vi "AlliGator Send Plots to Image Profile Window.vi"(7 "Image Control Refnum":T2, 8 "error in (no error)":errorcluster, 9 "Fit Parameter":T1, 11 "AlliGator IV DVR in":refnum<data-value>) -> (0 "error out":errorcluster, 3 "AlliGator IV DVR out":refnum<data-value>)   [LabVIEW 2021, in "AlliGator Image Profile Window.lvlib"]
doc: "Computes plots and send them to the Profile Window."
uses:
  AlliGator Image Profile Window.lvlib
  Internal Variables/AlliGator Internal Variables v2.ctl
  <vilib>/vision/Image Controls.llb/IMAQ Image.ctl
  Internal Variables/AlliGator Gate Image Set.ctl
  Files/AlliGator FLI Dataset Type.ctl
  Files/AlliGator Data Series Type.ctl
  Dual-Channel Datasets/AlliGator Dataset Channel.ctl
  Settings/AlliGator Gate Arithmetic.ctl
  Source Image/AlliGator Displayed Image.ctl
  Image/Named ROI Description.ctl
  Phasor Graph/AlliGator Decay Metadata v3.ctl
  Decay Analysis/Decay Preprocessing/AlliGator Decay Background Subtraction Info.ctl
  Decay Analysis/Decay Preprocessing/AlliGator Baseline Subtraction Method.ctl
  Graphs/XY Graph/XY Graph Plot Shift Parameters.ctl
  Graphs/XY Graph/XY Graph Plot Shift Method.ctl
  Decay Analysis/Decay Preprocessing/AlliGator Decay Extrapolation Parameters.ctl
  Phasor/Calibration Phasor (m, phi).ctl
  Phasor/Phasor Reference Series.ctl
  Phasor/Phasor Calibration Map v2.ctl
  Phasor/Phasor (g, s).ctl
  Phasor Graph/AlliGator Raw Phasor Plot Data v5.ctl
  Phasor/Phasor Standard Deviation Options.ctl
  Phasor Plot/AlliGator Phasor Multi-Harmonic Data.ctl
  Phasor/Phasor Harmonic Data.ctl
  Decay Fit Parameter Map/AlliGator Decay Fit Options & Parameters v4.ctl
  Fits/IRF(X)PSED/Decay Fit Options v4.ctl
  Fits/Decay Convolution/Decay Model.ctl
  Fits/Residual Type.ctl
  Fits/IRF(X)PSED/Fit Weights Type v2.ctl
  Fits/Non-linear Fitting Method v2.ctl
  Fits/Fit Calculation Method.ctl
  Fits/Non-linear Fitting Algorithm.ctl
  Decay Analysis/Decay Fit/AlliGator Decay Fit Parameter Constraints 2.ctl
  Fits/IRF(X)PSED/Decay Fit Parameters In List.ctl
  Fits/IRF(X)PSED/MLE Baseline Offset Type.ctl
  Decay Analysis/Decay Preprocessing/AlliGator Decay Preprocessing Parameters.ctl
  Fits/IRF(X)PSED/Decay Fit Parameters & Derived Quantities List v2.ctl
  Fits/IRF(X)PSED/Decay Fit Result Constraint.ctl
  Decay Fit Parameter Map/AlliGator Parameter Maps Data.ctl
  Image/Image Control Refnum.ctl
  Globals, Variables, Constants/AlliGator Variables List.ctl
  Settings/AlliGator Settings List.ctl
  Image/Box Profile Type.ctl
  AlliGator Image Profile Average Intensity Type.ctl
  AlliGator Image Profile Intensity Type.ctl
  AlliGator Image Profile Data.ctl
  Image/Image ROI Type.ctl
  AlliGator Image Profile Plot Data.ctl
  Graphs/XY Graph/XY Graph Plot Data.ctl
  Phasor/Phasor Ratio Type.ctl
  Phasor Ratio/AlliGator Phasor Ratio Color-Coded Quantity.ctl
  Variant/Variant to Data/Variant to Boolean.vi
  Variant/Variant to Data/Variant to DBL.vi
  Variant/Variant to Data/Variant to U16.vi
  Globals, Variables, Constants/AlliGator Globals, Variables & Constants.lvlib
  Graphs/XY Graph/XY Graph Add-Ons.lvlib
  Image/Image.lvlib
  Settings/AlliGator Settings.lvlib
  Variant/Variant to Data/Variant to Data.lvlib
  Decay Fit Parameter Map/AlliGator Decay Fit Parameter Map.lvlib
  Phasor/Phasor.lvlib
  Phasor Ratio/AlliGator Phasor Ratio.lvlib
  Math/Math.lvlib
  Internal Variables/AlliGator Internal Variables.lvlib
  Files/AlliGator Files.lvlib
  Phasor Graph/AlliGator Phasor Graph.lvlib
  Decay Analysis/Decay Preprocessing/AlliGator Decay Preprocessing.lvlib
  Phasor Plot/AlliGator Phasor Plot.lvlib
  Source Image/AlliGator Source Image.lvlib
  Fits/Fits.lvlib
  Decay Analysis/Decay Fit/AlliGator Decay Fit.lvlib
  Dual-Channel Datasets/AlliGator Dual-Channel Datasets.lvlib
panel:
  # "see the AlliGator License on the block diagram (Ctrl+E or Window:Show Block Diagram)"
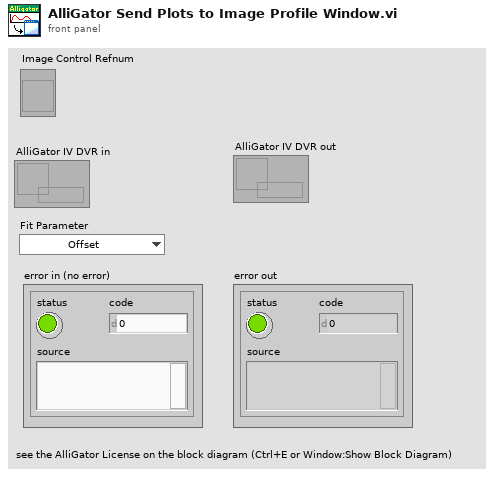
[diagram p1: front panel]
types:
  T1 = typedef "Fits.lvlib/Decay Fit Parameters & Derived Quantities List v2.ctl" = enum16{"Offset", "Baseline", "A_1", "tau_1", "A_2", "tau_2", "<tau>_a", "f1_a", "f2_a", "<tau>_i", "f1_i", "f2_i", "-", "R^2", "Chi^2"}
  T2 = typedef "Image.lvlib/Image Control Refnum.ctl" = refnum<vi>
  T3 = typedef "AlliGator Globals, Variables & Constants.lvlib/AlliGator Variables List.ctl" = enum16{"---- GUI ----", "GUI:Initialization Status", "GUI:State Indicators Refnum", "GUI:Original AlliGator Menu Items", "GUI:Current Action Loop State", "GUI:Script in progress", "GUI:Playback", "GUI:Loop Playback", "GUI:Search ROI Used", "GUI:Search ROI", "Decay Graph Max Legend Size", "Intensity Graph Max Legend Size", "Decay Statistics Graph Max Legend Size", "Phasor Graph Max Legend Size", "Phasor Ratio Graph Max Legend Size", "Lifetime Graph Max Legend Size", "---- Files ----", "Files:Export Dataset Frames as Individual Files", "Files:Show Batch Export Help Balloons", "Files:Frames in Dataset", "Files:ptu File Frame Start Indices", "Files:Current Frame in Dataset", "Files:Current Frame Timestamp", "Files:Dataset Loaded", "Files:Dataset Metadata", "Files:Dataset Channel", "Files:Dataset Data Description", "Files:Background Dataset Metadata", "Files:Background Dataset Channel", "Files:Background Dataset Data Description", "Files:Background File Subtraction", "Files:Background File Path", "Files:Background File Pile-up Correction", "Files:Background File Pixel Well Capacity", "Files:Background File Scaling Factor", "Files:Current Dataset Load Settings", "Files:Dataset Path", "Files:ICCD-specific Information", "Files:Macrotime Gate Separation", "------ Python Plugins ------", "Python Plugins:Information", "Python Plugins:Python Session", "Python Plugins:Valid Python Session?", "---- Source Image ----", "Source Image:ROIs", "Source Image:Current ROI", "Source Image:ROI Event Refnum", "X_Source Image:Display Range", "X_Source Image:Palette Information", "X_Source Image:Type of Displayed Image", "X_Time Gate Slider", "Source Image:Palette List", "Source Image:Scale", "Source Image:ROI Overlay Color", "Source Image:Overlay to Erase", "Source Image:Is Displayed Image Accumulated", "Source Image:White Light Image Modified", "Source Image:Mask Image Modified", "---- Image Profile Window ----", "Image Profile:Window Event Refnum", "Image Profile:IntensityType", "Image Profile:Intensity Average Type", "Image Profile:Intensity-weighted SDV", "Image Profile:Box Profile Type", "Image Profile:Window Open", "Image Profile:Plotted Fit Parameter", "------ Phasor Graph -------", "Phasor Graph:Show Line", "---- Phasor Plot ---", "Phasor Plot:Parameters Changed", "Phasor Plot:FLI Dataset Modified since last Calculation", "Phasor Harmonics Data", "Selected Phasor Harmonics", "Phasor Harmonic Manager Event Refnum", "Phasor Plot:ROIs", "Phasor Plot:Current ROI", "Phasor Plot:ROI Event Refnum", "Phasor Plot:Image Reference Points", "Phasor Plot:Computed", "Phasor Plot:Palette Information", "Phasor Plot:Palette List", "Phasor Plot:Phasor Ratio Palette Information", "Phasor Plot:Phasor Ratio Palette List", "Phasor Plot:Image Scale", "Phasor Plot:Image Overlay to Erase", "Phasor Plot:Image Elements to Update", "Phasor Plot:Current Calculation Parameters", "Phasor Plot:Current Calibration Options", "Phasor Plot:Reset Cumulated Phasor Plot", "Phasor Plot:Reference 1", "Phasor Plot:Lifetime Reference 1", "Phasor Plot:Reference 1 Frequency", "Phasor Plot:Reference 2", "Phasor Plot:Lifetime Reference 2", "Phasor Plot:Reference 2 Frequency", "---- Decay Analysis ----", "Number of Selected Decays to Fit", "LS Fit Results", "LAR Fit Results", "BS Fit Results", "Last Decay Max - Min", "Best Fit Parameters", "Best Fit Parameter Names", "Actual Size X", "Actual Size Y", "Binning X", "Binning Y", "Actual # Gates", "Dataset Number", "Gates to...", "Gates Skipped", "Gates to keep", "Gate Step", "Gate Separation", "Reversed Gates", "Pile-up Correction", "Pixel Well Capacity", "Background Subtracted", "Background Subtraction Method", "Background Definition Range", "Background File (deprecated)", "Number of Dataset Accumulated", "Array of Accumulated Dataset Paths", "Do Averaged Datasets", "Destination File Path", "Process Plot Target", "Use 1/D as Phasor Frequency", "---- Decay Fit Parameter Map -----", "Decay Fit Parameter Map:Palette Information", "Decay Fit Parameter Map:Palette List", "Decay Fit Parameter Map:X Resolution", "Decay Fit Parameter Map:Y Resolution", "Decay Fit Parameter Map:Use Decay Fit Result Constraints", "Decay Fit Parameter Map:Decay Fit Result Constraints", "Decay Fit Parameter Map:Decay Fit Result Constraints Applied", "---- Parameter Map ----", "Parameter Map:Palette Information", "Parameter Map:Palette List", "------- Local Decay Window ---------", "Local Decay Graph Window:Event Refnum", "Local Decay Graph Window:Use normalized IRF for convolution", "----- Miscellaneous ----", "Misc:Skippable Dialog Windows Status"}
  T4 = typedef "AlliGator Image Profile Window.lvlib/AlliGator Image Profile Intensity Type.ctl" = enum16{"Raw Data", "Displayed Image", "Background-subtracted"}
  T5 = typedef "AlliGator Image Profile Window.lvlib/AlliGator Image Profile Average Intensity Type.ctl" = enum16{"Integrated Intensity", "Average Intensity", "Intensity-weighted Average Intensity"}
  T6 = typedef "Image.lvlib/Box Profile Type.ctl" = enum16{"Full Width", "Half Width"}
  T7 = typedef "AlliGator Settings.lvlib/AlliGator Settings List.ctl" = enum16{"GUI:Visible Settings Tab", "GUI:Last Run Version", "Source Image:Use Image Histogram for Contrast", "Source Image:Low Count Pixels Rejection Options", "Source Image:High Count Pixels Rejection Options", "Source Image:Use Image Brightness", "Source Image:Blend Overlay with Image Background", "Source Image:Use Fixed ROI Diameter", "Source Image:ROI Diameter", "Source Image:ROI Center Color", "Source Image:Peak Threshold", "Source Image:Intensity Threshold", "Source Image:Image Binning Options", "Source Image:Image Smoothing Options", "Source Image:Image Histogram Active", "Source Image:Invert Binary Mask", "Source Image:Hot Pixel Removal", "Source Image:Overlay Analyzed ROI Center", "Source Image:Auto-Adjust Contrast", "Source Image:Histogram Lower Percentile", "Source Image:Histogram Upper Percentile", "Source Image:Save Source Image", "Source Image:Scale Bar Options", "Source Image:Image Resolution (Pixel Size)", "Source Image:Flatfield Correction", "Source Image:Show Dead Left Columns Correction", "Source Image:Dead Left Columns Correction", "Source Image:Image Pre-Processing Operations Order", "Source Image:Overlay ROI Median", "Source Image:Median Overlay Color", "Data Information:Gate Width", "Data Information:Nanotime Gate Separation", "Data Information:Macrotime Gate Separation", "Data Information:Gate Step", "Data Information:# Gates", "Data Information:Gate Image Exposure", "Data Information:Gate Image Integration", "Data Information:Gates to Skip", "Data Information:Gates to Keep", "Data Information:Define Gates to", "Data Information:Channel Name", "Data Information:Available Channel Names", "Data Information:Channel Arithmetic", "Data Information:Background File Subtraction", "Data Information:Background File", "Data Information:Background Scaling Factor", "Data Information:Background Pile-up Correction", "Data Information:Background Pixel Well Capacity", "Data Information:Laser Period", "Data Information:SYNC Period", "Data Information:Pile-up Correction", "Data Information:Pixel Well Capacity", "Data Information:Dataset Scaling Factor", "Fluorescence Decay_Decay Pre-Processing:Reverse Gates", "Fluorescence Decay_Decay Pre-Processing:Verbose Decay Pre-Processing", "Fluorescence Decay_Decay Pre-Processing:Use Decay Pre-Processing", "Fluorescence Decay_Decay Pre-Processing:Background Subtraction", "Fluorescence Decay_Decay Pre-Processing:Background Definition Range", "Fluorescence Decay_Decay Pre-Processing:Baseline Subtraction Method", "Fluorescence Decay_Decay Pre-Processing:Decay Pre-Processing Operations Order", "Fluorescence Decay_Decay Pre-Processing:Smoothing Parameter", "Fluorescence Decay_Decay Pre-Processing:Shift Decay", "Fluorescence Decay_Decay Pre-Processing:Decay Shift Parameters", "Fluorescence Decay_Decay Pre-Processing:Fold Decay", "Fluorescence Decay_Decay Pre-Processing:# Folds", "Fluorescence Decay_Decay Pre-Processing:1-Normalize Decay", "Fluorescence Decay_Decay Pre-Processing:[0-1]-Normalize Decay", "Fluorescence Decay_Decay Pre-Processing:Smoothen Decay", "Fluorescence Decay_Decay Pre-Processing:Extrapolate Decay", "Fluorescence Decay_Decay Pre-Processing:Use Periodicity", "Fluorescence Decay_Decay Pre-Processing:Use Cursors", "Fluorescence Decay_Decay Pre-Processing:Tail Fraction", "Fluorescence Decay_Decay Pre-Processing:Head Fraction", "Fluorescence Decay_Decay Pre-Processing:Additional Points", "Fluorescence Decay_Decay Pre-Processing:Straighten Decay", "Fluorescence Decay_Decay Pre-Processing:Constant Background", "Fluorescence Decay_Decay Pre-Processing:Pixel-Normalize Decay", "Fluorescence Decay_Advanced Analysis:Extract IRF instead of Decay", "Fluorescence Decay_Advanced Analysis:IRF Extraction Options", "Fluorescence Decay_Advanced Analysis:IRF Optimization Options", "Fluorescence Decay_Advanced Analysis:Square Pulse Options", "Fluorescence Decay_Advanced Analysis:IRF Order", "Fluorescence Decay_Advanced Analysis:IRF Time Constants", "Fluorescence Decay_Advanced Analysis:Wavelet Analysis Options", "Fluorescence Decay_Advanced Analysis:Average Lifetime Options", "Fluorescence Decay_Fit Options:Fit Options", "Fluorescence Decay_Fit Options:Use Legacy Fitting Approach", "Fluorescence Decay_Fit Options:Use Data Information Laser Period", "Fluorescence Decay_Fit Parameters:Displayed Fit Parameters", "Fluorescence Decay_Fit Parameters:Fit Parameter Constraints", "Fluorescence Decay_Fit Parameters:Export Tabulated Results", "Fluorescence Decay_Fit Parameters:MLE Baseline Offset Type", "Fluorescence Decay_Fit Parameters:MLE Baseline Offset", "Fluorescence Decay_Fit Parameters:Guess Parameter Names", "Fluorescence Decay_Fit Parameters:Guess Parameter Values", "Fluorescence Decay_Fit Parameters:Guess Parameters Options", "Fluorescence Decay_Fit Parameters:Optimal Offset Selection Criterion", "Fluorescence Decay_Styles:Show Last Decay Only", "Fluorescence Decay_Styles:Decay Graph Color Array", "Fluorescence Decay:Decay Graph Active", "Fluorescence Decay Statistics:Min Peak Value", "Fluorescence Decay Statistics:Reject Low Decay Peak Pixels", "Fluorescence Decay Statistics:Reject High Decay Peak Pixels", "Fluorescence Decay Statistics:Max Peak Value", "Time Traces:Use File Timestamp", "Time Traces:Time Step", "Time Traces:Use Intensity Correction File", "Time Traces:Intensity Correction File", "Phasor Plot:Phasor Plot Smoothing Options", "Phasor Plot:Phasor Plot Size", "Phasor Plot:Phasor Plot Graphics Options", "Phasor Plot:Cumulative Phasor Plot", "Phasor Plot:Use Phasor Brightness", "Phasor Plot:Blend Overlay with Phasor Background", "Phasor Plot:Save Phasor Plot", "Phasor Plot:Show References", "Phasor Plot:Phasor Ratio Decay Range", "Phasor Plot:Exponential Fading", "Phasor Plot:Phasor Ratio Reference Colors", "Phasor Plot:Reference Radius", "Phasor Plot:Show Color Map Vertices", "Phasor Plot:Phasor Plot Active", "Phasor Plot:Phasor Ratio Color Map Type", "Phasor Plot:Phasor Ratio Color Map", "Phasor Plot:Phasor Ratio Display Range", "Phasor Plot:Selected Image ROI(s)", "Phasor Plot:All Image ROIs", "Phasor Plot:Selected Phasor Plot ROI(s)", "Phasor Plot:All Phasor Plot ROIs", "Phasor Plot:Phasor Ratio Color-Coded Quantity", "Phasor Plot:Store Phasor Harmonics", "Phasor Plot:Draw Reference Segment", "Phasor Plot:User-Defined Quantity", "Phasor Plot:Color Scale High Color", "Phasor Plot:Color Scale Low Color", "Phasor Plot:Intensity-weighted Phasor Plot", "Phasor Graph:Phasor Frequency", "Phasor Graph:Phasor Ratio Type", "Phasor Graph:Pixel-level Phasor Computation", "Phasor Graph:Save Phasor Graph", "Phasor Graph:Phasor Graph Active", "Phasor Graph:Phasor SDV Options", "Phasor Graph:Intensity-weighted Phasor Graph", "Phasor Graph:Define Shortest Lifetime as", "Phasor Calibration:Use Backup Calibration if needed", "Phasor Calibration:Backup Calibration Type", "Phasor Calibration:Calibration Type", "Phasor Calibration:Calibration Lifetime", "Phasor Calibration:Calibration Map Algorithm", "Single-Exponential Phasor Locus (SEPL):Gate Parameters", "Single-Exponential Phasor Locus (SEPL):User-defined Gate", "Single-Exponential Phasor Locus (SEPL):User-defined IRF", "Single-Exponential Phasor Locus (SEPL):Phasor Parameters", "Single-Exponential Phasor Locus (SEPL):Decay & IRF Parameters", "Single-Exponential Phasor Locus (SEPL):Display Parameters", "Lifetime Analysis:Decay Analysis Parameters", "Lifetime Analysis:Lifetime Map Active", "Plugins:Python Settings", "Miscellaneous:Verbose Mode", "Miscellaneous:Beep after Script", "Miscellaneous:Saved Image File Format", "Miscellaneous:Exported Gate Image Settings", "Miscellaneous:Include Loading in Timing", "Miscellaneous:Verbose Settings Mode", "Miscellaneous:Histogram Options", "Miscellaneous:Beep on Error", "Miscellaneous:# Logical Processors Used", "Miscellaneous:ROI Description Max Characters", "Miscellaneous:Verbose Error Mode", "Miscellaneous:Transparent Mask Color"}
  T8 = typedef "AlliGator Image Profile Window.lvlib/AlliGator Image Profile Data.ctl" = cluster{"ROI Type":T9, "End Points":cluster{"X":dbl, "Y":dbl}[], "Profile Data":T10[]}
  T9 = typedef "Image.lvlib/Image ROI Type.ctl" = enum16{"No Selection", "Point", "Line", "Rectangle", "Oval", "Polygon", "Freehand Region", "Annulus", "Unused2", "Unused3", "Broken Line", "Freehand Line", "Rotated Rectangle"}
  T10 = typedef "AlliGator Image Profile Window.lvlib/AlliGator Image Profile Plot Data.ctl" = cluster{"Plot Name":string, "Plot":T11}
  T11 = typedef "XY Graph Add-Ons.lvlib/XY Graph Plot Data.ctl" = cluster{"X Array":dbl[], "Y Array":dbl[]}
  T12 = typedef "AlliGator Phasor Ratio.lvlib/AlliGator Phasor Ratio Color-Coded Quantity.ctl" = enum16{"Phasor Ratio (f1 or a1)", "Average Lifetime (<tau>_i or <tau>_a))", "User-Defined Quantity"}
  T13 = typedef "Phasor.lvlib/Phasor Ratio Type.ctl" = enum32{"Intensity-weighted", "Amplitude-weighted"}
  T14 = typedef "AlliGator Internal Variables.lvlib/AlliGator Internal Variables v2.ctl" = cluster{"----------------------------- Images -----------------------------":u8, "Displayed Image":T15, "White Light Image":T15, "Mask Image":T15, "ROI Mask Image":T15, "Current Dataset Images 1":T16, "Background Dataset Images 1":T16, "Current Dataset Images 2":T16, "Background Dataset Images 2":T16, "Current Dataset Arithmetic Images":T16, "Accumulated Dataset Images 1":T16, "Accumulated Dataset Images 2":T16, "Accumulated Dataset Arithmetic Images":T16, "----------------------------- File Paths -----------------------------":u8, "Phasor Plot Image":T15, "Decay Fit Parameter Map Image":T15, "Parameter Map Image":T15, "Single Data Point Path":path, "White Light Image Path":path, "Mask Image Path":path, "Time-Series Folder":path, "[Time-Series Paths]":path[], "----------------------------- FLI Dataset -----------------------------":u8, "Current Dataset":i32, "Single Dataset Type":T17, "Current Folder":string, "AlliGator Data Series Type":T18, "# Datasets":i32, "Dual-Channel Dataset":bool, "Selected Channel Name":string, "Dataset Channel":T19, "Channel Arithmetic":T20, "Dual-Channel Background Dataset":bool, "Background Channel":T19, "Dual-Channel Accumulated Dataset":bool, "Start Time":dbl, "[Time-Series Timestamps]":dbl[], "[Intensity Corrections]":dbl[], "Time Series Script":bool, "Type of Displayed Image":T21, "Gate Image Slide":u16, "# Gates":i32, "ROIs":T22[], "----------------------------- Decays -----------------------------":u8, "ROI Decay":cluster{"t Array":dbl[], "I Array":dbl[]}, "Valid Decay":bool, "Decay  Metadata":T24, "Reference Decay Plot Name":string, "Reference Decay":cluster{"t Array":dbl[], "I Array":dbl[]}, "Decay Shift Plot":cluster{"Time Stamps":dbl[], "Decay Shifts":dbl[]}, "[Decays Max Values]":sgl[], "[Decays Min Values]":sgl[], "----------------------------- Calibration -----------------------------":u8, "Calibration Phasor":T30, "Calibration Phasor Series":T31, "Phasor Calibration Map":T32, "Calibration Map MD5 Digest":string, "----------------------------- Phasor Graph -----------------------------":u8, "Last Raw Phasor":T33, "Last Calibrated Phasor":T33, "Last Calibrated Phasor SDV":T33, "Phasor Graph:Phasor Plot":cluster{"g Array":dbl[], "s Array":dbl[]}, "Phasor Graph:Phasor SDV Plot":cluster{"g Array":dbl[], "s Array":dbl[]}, "[Phasor Graph:Raw Phasor Plots]":T34[], "Phasor Plot locked to Ref 1":i32, "[Phasor Plot(s) locked to Ref 1]":i32[], "[Phasor Plot(s) locked to Ref 2]":i32[], "[Pixel Phasors]":T33[], "----------------------------- Phasor Plot -----------------------------":u8, "[[Sum Image]]":dbl[][], "[[CSG Phasors]]":csg[][], "[[Valid Pixel?]]":bool[][], "[[Phasor Ratios]]":dbl[][], "[[Average Lifetimes]]":dbl[][], "Amplitude Weighted Average Lifetime":bool, "I/m/phi Dataset":cluster{"I/m/phi Dataset?":bool, "Base Frequency":dbl[unit], "Harmonic Orders":u8[]}, "Multi Phasor Plot Data":T36, "----------------------------- Decay Fit Parameter Map -----------------------------":u8, "Decay Fit Options & Parameters":T38, "Fit Options: Decay Preprocessing Parameters":T49, "Fit Options: Reference Decay":cluster{"t Array":dbl[], "I Array":dbl[]}, "Is Full Image Parameters Map":bool, "Is Single-Pixels Parameters Map":bool, "NLSF Parameters Map X Resolution":i32, "NLSF Parameters Map Y Resolution":i32, "[Single Decay Fit Parameters]":dbl[], "Fit Model":T40, "[[Multiple Decays Fit Parameters]]":dbl[][], "[[Multiple Decays Fit Parameter SDVs]]":dbl[][], "[[IRFs]]":dbl[][], "[ROI Descriptors]":T23[], "IRF Array Time Axis":dbl[], "Decay Array Time Axis":dbl[], "[Decay Fit Parameter Names]":T1[], "[Decay Sum]":dbl[], "Array of Decay Fit Result Constraints":T50[], "Selected ROIs Array":bool[], "----------------------------- Parameter Maps -----------------------------":u8, "[Map Set Names]":string[], "[Parameter Maps]":T51[], "[[User-defined Quantities]]":dbl[][], "User-defined Quantity":string}
  T15 = typedef "IMAQ Image.ctl" = refnum<image>
  T16 = typedef "AlliGator Internal Variables.lvlib/AlliGator Gate Image Set.ctl" = cluster{"SGL Gate Images":T15[], "SGL Sum Image":T15, "SGL Max Image":T15, "SGL Min Image":T15}
  T17 = typedef "AlliGator Files.lvlib/AlliGator FLI Dataset Type.ctl" = enum16{"HDF5 FLI Dataset", "Gate Image Folder", ".sdt FLI Dataset (Becker & Hickl)", ".ptu FLI Dataset (PicoQuant)", "SS1 FLI Dataset", "SS2 FLI Dataset", "I/m/phi Dataset", ".bin FLI Dataset (PicoQuant Binned)", ".bin FLI Dataset (Piccolo Binned)", ".mat FLI Dataset"}
  T18 = typedef "AlliGator Files.lvlib/AlliGator Data Series Type.ctl" = enum16{"Not a Supported Series", "Gate Images Folder Series", "SwissSPAD 2 Dataset Series", "B&H FLI Dataset Series", "PicoQuant PTU FLI Dataset Series", "PicoQuant BIN FLI Dataset Series", "Piccolo hist BIN FLI Dataset Series", "HDF5 FLI Dataset Series"}
  T19 = typedef "AlliGator Dual-Channel Datasets.lvlib/AlliGator Dataset Channel.ctl" = enum16{"G2", "INT"}
  T20 = typedef "AlliGator Settings.lvlib/AlliGator Gate Arithmetic.ctl" = enum16{"None", "INT-G2", "G2/INT*<INT>", "(1 - G2/INT)*<INT>"}
  T21 = typedef "AlliGator Source Image.lvlib/AlliGator Displayed Image.ctl" = enum16{"Single Gate", "Sum of All Gates", "Max of All Gates", "Min of All Gates", "-", "White Ligth Image", "Mask Image"}
  T22 = typedef "Image.lvlib/Named ROI Description.ctl" = cluster{"ROI Descriptor":T23, "ROI Name":string, "Overlay Color":u32}
  T23 = typedef "ROI Descriptor" = cluster{"Global Rectangle":i32[], "Contours":cluster{"ID":enum32{"External", "Internal"}, "Type":u32, "Coordinates":i32[]}[]}
  T24 = typedef "AlliGator Phasor Graph.lvlib/AlliGator Decay Metadata v3.ctl" = cluster{"ROI Descriptor":T23, "ROI Center":cluster{"X":i32, "Y":i32}, "Decay Background Subtraction Info":T25, "Decay Reverted":bool, "Decay Smoothened":bool, "Decay Straightened":bool, "Fitted Tau (Decay Straightening)":dbl, "Decay Shift Parameters":T27, "Decay Shifted":bool, "Decay Extrapolated":bool, "Decay Extrapolation Parameters":T29, "Decay Normalized":bool, "Fold Decay":bool, "# Folds":u32}
  T25 = typedef "AlliGator Decay Preprocessing.lvlib/AlliGator Decay Background Subtraction Info.ctl" = cluster{"Laser Period":dbl[unit], "Gate Duration":dbl[unit], "Baseline Subtraction Method":T26, "Background Definition Range":cluster{"Min Gate":dbl[unit], "Max Gate":dbl[unit]}, "Total Intensity w/o Bkgd Subtraction":dbl, "Bkgd-subtracted Intensity (exp)":dbl, "# Data Points":i32, "Background/Gate":dbl, "Fitted Lifetime":dbl[unit], "Bkgd-subtracted Intensity (theo)":dbl}
  T26 = typedef "AlliGator Decay Preprocessing.lvlib/AlliGator Baseline Subtraction Method.ctl" = enum16{"Mean", "Min", "Square Gated Single-Exponential", "File", "Constant"}
  T27 = typedef "XY Graph Add-Ons.lvlib/XY Graph Plot Shift Parameters.ctl" = cluster{"Type":T28, "Shift":dbl[unit], "Threshold":dbl, "Rotate":bool}
  T28 = typedef "XY Graph Add-Ons.lvlib/XY Graph Plot Shift Method.ctl" = enum16{"Default", "CFD", "Threshold", "Cross-Correlation"}
  T29 = typedef "AlliGator Decay Preprocessing.lvlib/AlliGator Decay Extrapolation Parameters.ctl" = cluster{"Additional Points":u32, "Head Fraction":dbl, "Fitted Tau":dbl, "Use Periodicity":bool, "Use Cursors":bool, "Tail Fraction":dbl}
  T30 = typedef "Phasor.lvlib/Calibration Phasor (m, phi).ctl" = cluster{"m":dbl, "phi":dbl, "Phasor Frequency":dbl[unit], "Reference Lifetime":dbl[unit]}
  T31 = typedef "Phasor.lvlib/Phasor Reference Series.ctl" = cluster{"m Array":dbl[], "phi Array":dbl[], "Phasor Frequency":dbl[unit], "Calibration Lifetime":dbl[unit]}
  T32 = typedef "Phasor.lvlib/Phasor Calibration Map v2.ctl" = cluster{"Phasor Frequency":dbl[unit], "Calibration Lifetime":dbl[unit], "ROI Centers":cluster{"X":i32, "Y":i32}[], "ROI Descriptors":T23[], "Map Resolution X":i32, "Map Resolution Y":i32, "z Array":cdb[]}
  T33 = typedef "Phasor.lvlib/Phasor (g, s).ctl" = cluster{"g":dbl, "s":dbl}
  T34 = typedef "AlliGator Phasor Graph.lvlib/AlliGator Raw Phasor Plot Data v5.ctl" = cluster{"Phasor Plot Name":string, "Raw Phasor Plot":T33[], "Phasor Frequency":dbl[unit], "[Decay Metadata]":T24[], "Raw Phasor Plot SDV":T33[], "Phasor SDV Options":T35, "[Calibration Phasor]":T30[], "Intensity Array":dbl[]}
  T35 = typedef "Phasor.lvlib/Phasor Standard Deviation Options.ctl" = cluster{"Compute Estimated SDV":bool, "# Replicas":u32, "Use Estimated Average Phasor":bool}
  T36 = typedef "AlliGator Phasor Plot.lvlib/AlliGator Phasor Multi-Harmonic Data.ctl" = cluster{"Base Frequency":dbl[unit], "# Harmonics":u8, "Harmonic Orders":u8[], "Phasor Plot Settings Checksum":u64, "Phasor Harmonic Data Array":T37[]}
  T37 = typedef "Phasor.lvlib/Phasor Harmonic Data.ctl" = cluster{"Phasor Harmonic Name":string, "Phasor Plot Settings Checksum":u64, "Phasor Frequency":dbl[unit], "Base Frequency":dbl[unit], "Harmonic Order":u8, "Phasor Plot Parameters":string, "Phasor Array [[CSG]]":csg[][], "Dataset File Path":path}
  T38 = typedef "AlliGator Decay Fit Parameter Map.lvlib/AlliGator Decay Fit Options & Parameters v4.ctl" = cluster{"SYNC Period":dbl[unit], "Fit Options":T39, "Fit Parameter Constraints":T46[], "MLE Baseline Offset":dbl, "MLE Baseline Offset Type":T48}
  T39 = typedef "Fits.lvlib/Decay Fit Options v4.ctl" = cluster{"Show Fit Residuals":bool, "Fit Model":T40, "Residual Type":T41, "Max Decay Percentile":dbl, "Min Decay Percentile":dbl, "Show Full Decay":bool, "Weights":T42, "Fitting Method":T43, "Compute Parameter Uncertainties":bool, "Periodic Boundaries":bool, "Model Calculation":T44, "Period":dbl[unit], "Termination Criteria":cluster{"Max Iterations":i32, "Max Function Calls":i32, "Max Time":dbl[unit], "Function Tolerance":dbl, "Parameter Tolerance":dbl, "Gradient Tolerance":dbl, "Min Lambda":dbl, "Max Lambda":dbl, "Initial Tick Count":u32}, "Offset Resolution":dbl[unit], "Use Local IRF":bool, "Fitting Algorithm":T45, "Show Confidence Interval ":bool, "Confidence Level":dbl}
  T40 = typedef "Fits.lvlib/Decay Model.ctl" = enum16{"1-Exponential", "2-Exponentials"}
  T41 = typedef "Fits.lvlib/Residual Type.ctl" = enum16{"Standard", "Normalized", "Reduced"}
  T42 = typedef "Fits.lvlib/Fit Weights Type v2.ctl" = enum16{"Unweighted", "1/Variance (Neyman)", "1/Variance (Pearson)", "Best of All"}
  T43 = typedef "Fits.lvlib/Non-linear Fitting Method v2.ctl" = enum16{"Least Square", "Least Absolute Residual", "Bisquare", "MLE", "-", "Best of All"}
  T44 = typedef "Fits.lvlib/Fit Calculation Method.ctl" = enum16{"Simulation", "Convolution", "Integration"}
  T45 = typedef "Fits.lvlib/Non-linear Fitting Algorithm.ctl" = enum16{"Levenberg-Marquardt", "Trust-Region Dogleg"}
  T46 = typedef "AlliGator Decay Fit.lvlib/AlliGator Decay Fit Parameter Constraints 2.ctl" = cluster{"Fit Parameter":T47, "Min Value":dbl, "Max Value":dbl, "Global":bool, "Used":bool}
  T47 = typedef "Fits.lvlib/Decay Fit Parameters In List.ctl" = enum16{"Offset", "Baseline", "A_1", "tau_1", "A_2", "tau_2"}
  T48 = typedef "Fits.lvlib/MLE Baseline Offset Type.ctl" = enum32{"Absolute", "Percentage"}
  T49 = typedef "AlliGator Decay Preprocessing.lvlib/AlliGator Decay Preprocessing Parameters.ctl" = cluster{"Background Subtraction":bool, "Straighten Decay":bool, "Reverse Gates":bool, "1-Normalized Decay":bool, "Smoothen Decay":bool, "Smoothing Parameter":dbl, "Shift Decay":bool, "Decay Shift Parameters":T27, "Extrapolate Decay":bool, "Additional Points":u32, "Head Fraction":dbl, "Pixel-Normalize Decay":bool, "Use Periodicity":bool, "Use Cursors":bool, "Tail Fraction":dbl, "Use Decay Pre-Processing":bool, "Fold Decay":bool, "# Folds":u32, "[0-1]-Normalized Decay":bool}
  T50 = typedef "Fits.lvlib/Decay Fit Result Constraint.ctl" = cluster{"Fit Parameter":enum16{"Offset", "Baseline", "A_1", "tau_1", "A_2", "tau_2", "<tau>_a", "f1_a", "f2_a", "<tau>_i", "f1_i", "f2_i", "-", "R^2", "Chi^2", "Max Relative Residual", "<Residual ACF>", "Residual ACF SDV", "tau_2/tau_1"}, "Min Value":dbl, "Max Value":dbl, "Use Constraint":bool}
  T51 = typedef "AlliGator Decay Fit Parameter Map.lvlib/AlliGator Parameter Maps Data.ctl" = cluster{"Map Set Name":string, "[Parameter Names]":string[], "[[Parameters]]":dbl[][], "[[Parameter SDVs]]":dbl[][], "Decay Array Time Axis":dbl[], "[[IRFs]]":dbl[][], "IRF Array Time Axis":dbl[], "X Resolution":i32, "Y Resolution":i32, "Intensity Array":dbl[]}
  T52 = cluster{"Global Rectangle":i32[], "Contours":cluster{"Contour Type":u32, "ROI Type":u32, "Points":i32[]}[]}
  T53 = cluster{"Contour Type":u32, "ROI Type":u32, "Points":i32[]}[]
  T54 = cluster{"Contour Type":u32, "ROI Type":u32, "Points":i32[]}
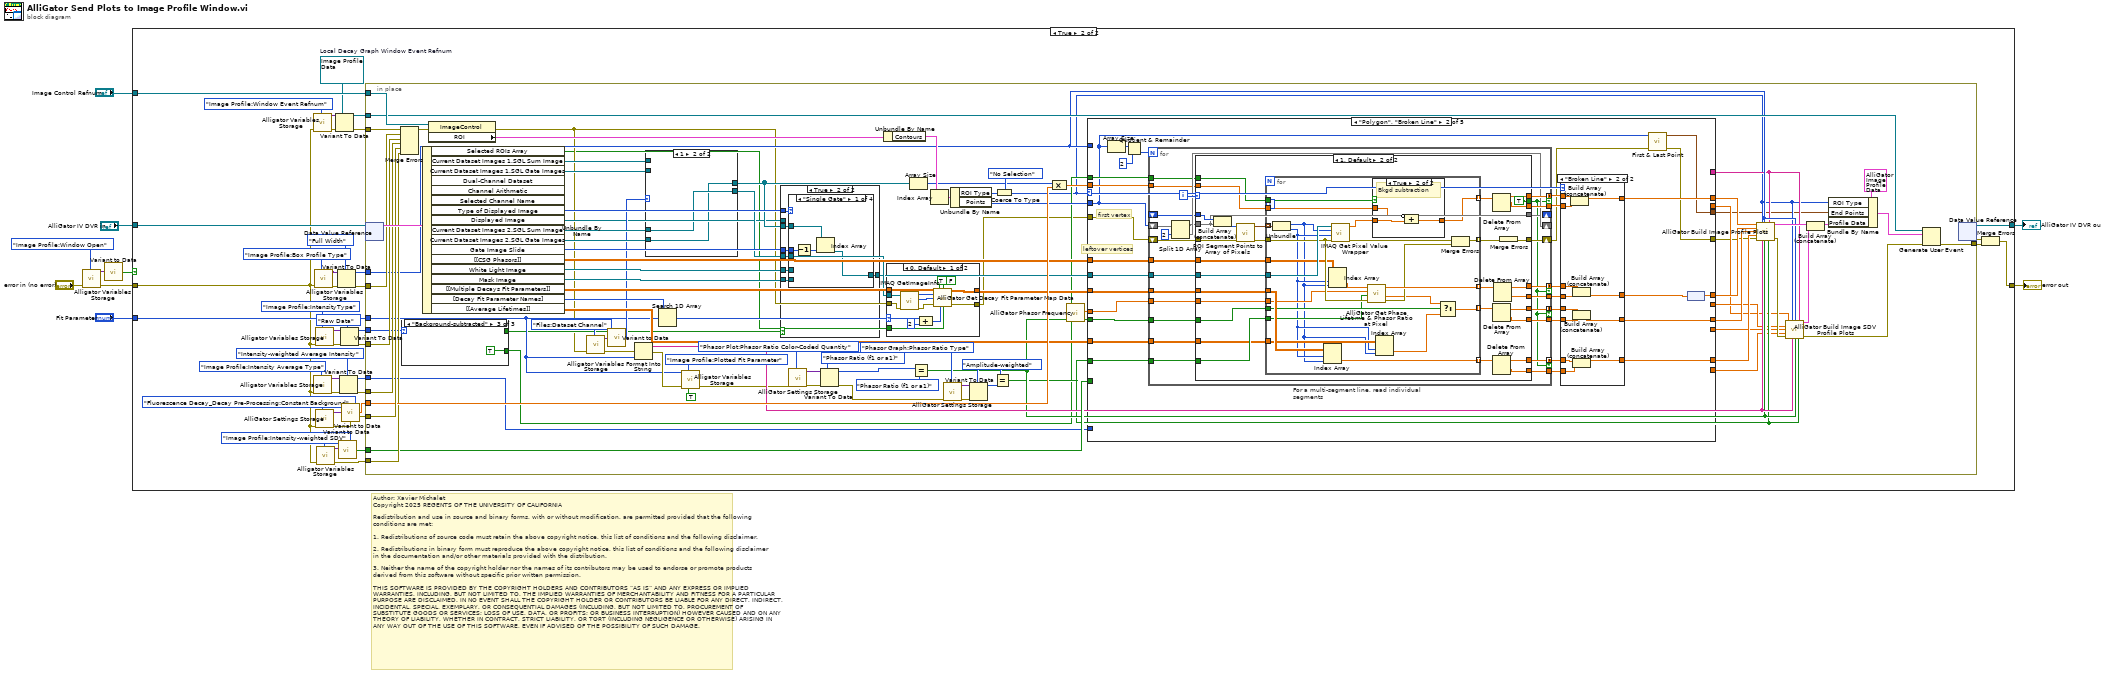
[diagram p0: block diagram]
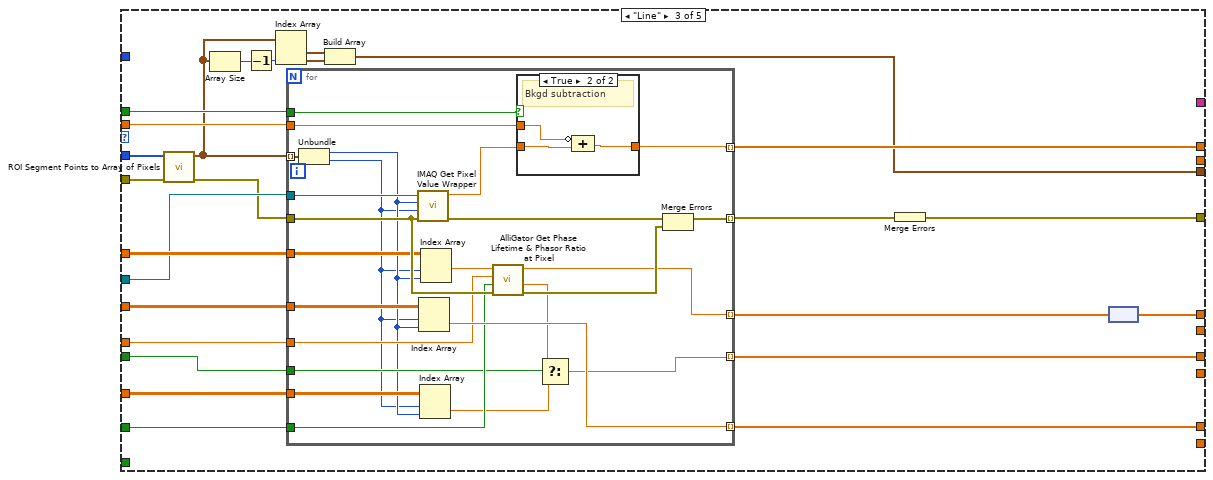
[diagram p7: hidden frame]
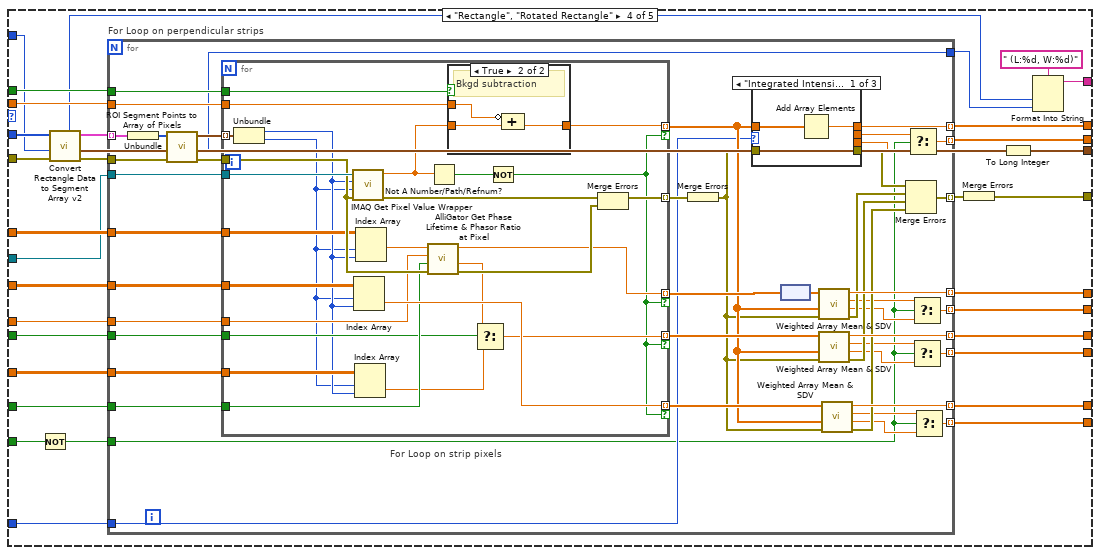
[diagram p9: hidden frame]
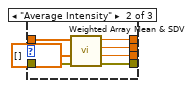
[diagram p10: hidden frame]
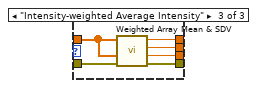
[diagram p11: hidden frame]
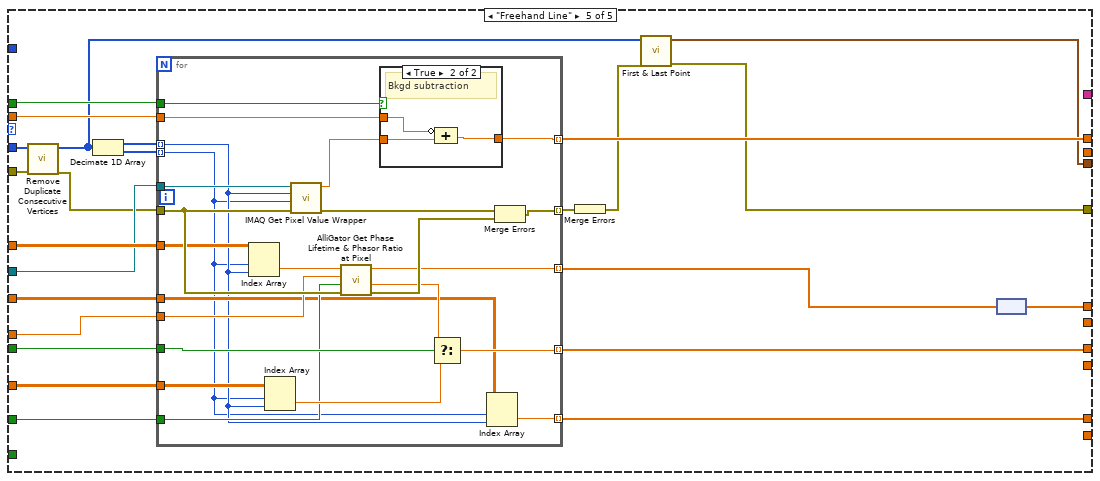
[diagram p13: hidden frame]
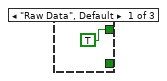
[diagram p15: hidden frame]
diagram:
  # "Author: Xavier Michalet\nCopyright 2025 REGENTS OF THE UNIVERSITY OF CALIFORNIA\n\nRedistribution and use in source and binary forms, with or without modification, are permitted provided that the following conditions are met:\n\n1. Redistributions of source code must retain the above copyright notice, this list of conditions and the following disclaimer.\n\n2. Redistributions in binary form must reproduce the above copyright notice, this list of conditions and the following disclaimer in the documentation and/or other materials provided with the distribution.\n\n3. Neither the name of the copyright holder nor the names of its contributors may be used to endorse or promote products derived from this software without specific prior written permission.\n\nTHIS SOFTWARE IS PROVIDED BY THE COPYRIGHT HOLDERS AND CONTRIBUTORS “AS IS” AND ANY EXPRESS OR IMPLIED WARRANTIES, INCLUDING, BUT NOT LIMITED TO, THE IMPLIED WARRANTIES OF MERCHANTABILITY AND FITNESS FOR A PARTICULAR PURPOSE ARE DISCLAIMED. IN NO EVENT SHALL THE COPYRIGHT HOLDER OR CONTRIBUTORS BE LIABLE FOR ANY DIRECT, INDIRECT, INCIDENTAL, SPECIAL, EXEMPLARY, OR CONSEQUENTIAL DAMAGES (INCLUDING, BUT NOT LIMITED TO, PROCUREMENT OF SUBSTITUTE GOODS OR SERVICES; LOSS OF USE, DATA, OR PROFITS; OR BUSINESS INTERRUPTION) HOWEVER CAUSED AND ON ANY THEORY OF LIABILITY, WHETHER IN CONTRACT, STRICT LIABILITY, OR TORT (INCLUDING NEGLIGENCE OR OTHERWISE) ARISING IN ANY WAY OUT OF THE USE OF THIS SOFTWARE, EVEN IF ADVISED OF THE POSSIBILITY OF SUCH DAMAGE."
  n1 = call "Alligator Variables Storage.vi"("AlliGator Variable"=AlliGator_Variables_List."Image Profile:Window Open" ("Alligator Variable"), "Error In"="error in (no error)") -> ("Error Out"=w2:errorcluster, "Data out"=w5:variant)  [unwired: 7 in, 1 out]
  n2 = call-poly "Variant to Data.vi"("Variant"=w5) -> ("Value"=w1:bool)  [unwired: 8 in]
  n3 = case shown="True" w1 {
    tunnel: "AlliGator IV DVR in" -> [w12 w52]
    tunnel: [w12 w51] -> w9
    tunnel: "Image Control Refnum" -> [_ w50]
    tunnel: [w11 w43] -> w7
    tunnel: "Fit Parameter" -> [_ w41]
    tunnel: w2 -> [w11 w24]
    frame False {
      # "Don't process data if the Image PRofile Window is not open"
    }
    frame True {
      w13 = refnum<user-event> refnum  # Local Decay Graph Window Event Refnum
      n4 = call "Alligator Variables Storage.vi"("AlliGator Variable"=AlliGator_Variables_List."Image Profile:Window Event Refnum" ("Alligator Variable"), "Error In"=w24) -> ("Error Out"=w48:errorcluster, "Data out"=w46:variant)  [unwired: 7 in, 1 out]
      n5 = call "Alligator Variables Storage.vi"("AlliGator Variable"=AlliGator_Variables_List."Image Profile:Intensity Average Type" ("Alligator Variable"), "Error In"=w24) -> ("Error Out"=w19:errorcluster, "Data out"=w20:variant)  [unwired: 7 in, 1 out]
      n6 = call "Alligator Variables Storage.vi"("AlliGator Variable"=AlliGator_Variables_List."Image Profile:Box Profile Type" ("Alligator Variable"), "Error In"=w24) -> ("Error Out"=w33:errorcluster, "Data out"=w34:variant)  [unwired: 7 in, 1 out]
      n7 = call "Alligator Variables Storage.vi"("AlliGator Variable"=AlliGator_Variables_List."Image Profile:IntensityType" ("Alligator Variable"), "Error In"=w24) -> ("Error Out"=w23:errorcluster, "Data out"=w21:variant)  [unwired: 7 in, 1 out]
      n8 = call "AlliGator Settings Storage.vi"("AlliGator Settings List"=AlliGator_Settings_List."Fluorescence Decay_Decay Pre-Processing:Constant Background", "Error In"=w24) -> ("Error Out"=w39:errorcluster, "Variant Data out"=w37:variant)  [unwired: 8 in]
      n9 = call "Alligator Variables Storage.vi"("AlliGator Variable"=AlliGator_Variables_List."Image Profile:Intensity-weighted SDV" ("Alligator Variable"), "Error In"=w24) -> ("Error Out"=w27:errorcluster, "Data out"=w26:variant)  [unwired: 7 in, 1 out]
      n10 = Variant To Data(error in=w48, type=w13, Variant=w46) -> (data=w45:refnum<user-event>, error out=w47:errorcluster)
      n11 = Variant To Data(error in=w33, type=Box_Profile_Type."Full Width" ("Box Profile Type"), Variant=w34) -> (data=w31:T6, error out=w30:errorcluster)
      n12 = call-poly "Variant to Data.vi"("Variant"=w26) -> ("Value"=w28:bool)  [unwired: 8 in]
      n13 = Variant To Data(error in=w19, type=AlliGator_Image_Profile_Average_Intensity_Type."Intensity-weighted Average Intensity" ("Image Profile Average Intenisty Type"), Variant=w20) -> (data=w14:T5, error out=w18:errorcluster)
      n14 = Variant To Data(error in=w23, type=AlliGator_Image_Profile_Intensity_Type."Raw Data" ("Image Profile Intensity Type"), Variant=w21) -> (data=w16:T4, error out=w22:errorcluster)
      n15 = call-poly "Variant to Data.vi"("Variant"=w37) -> ("Value"=w36:dbl)  [unwired: 8 in]
      n16 = in-place {
        in-place-border: w50 -> [w142]
        in-place-border: w47 -> [w141]
        in-place-border: w45 -> [w140]
        in-place-border: w41 -> [w71]
        in-place-border: w22 -> [w138]
        in-place-border: w18 -> [w137]
        in-place-border: w39 -> [w136]
        in-place-border: w36 -> [w135]
        in-place-border: w31 -> [w65]
        in-place-border: w30 -> [w134]
        in-place-border: [w87] -> w29
        in-place-border: w27 -> [w85]
        in-place-border: w28 -> [w84]
        in-place-border: w16 -> [w69]
        in-place-border: w14 -> [w66]
        w110 = Phasor_Ratio_Type."Amplitude-weighted" ("Phasor Ratio Type")
        n17 = in-place-dvr #1(w52) -> (w143:T14)  [unwired: 1 out]
        n18 = Merge Errors(w141, w134, w138, w137, w136, w85) -> (w139:errorcluster)
        n19 = case shown="\"Background-subtracted\"" w69 {
          tunnel: [TRUE ("Get(F)/Set") _ _] -> w68
          tunnel: [_ _ TRUE ("Get(F)/Set")] -> w67
          frame "Raw Data", Default {
          }
          frame "Displayed Image" {
          }
          frame "Background-subtracted" {
          }
        }
        n20 = Unbundle By Name(w143) -> ("Selected ROIs Array"=w53:bool[], "Current Dataset Images 1.SGL Sum Image"=w113:T15, "Current Dataset Images 1.SGL Gate Images"=w112:T15[], "Type of Displayed Image"=w125:T21, "Displayed Image"=w62:T15, "Current Dataset Images 2.SGL Sum Image"=w114:T15, "Current Dataset Images 2.SGL Gate Images"=w115:T15[], "Gate Image Slide"=w124:u16, "[[CSG Phasors]]"=w126:csg[][], "White Light Image"=w123:T15, "Mask Image"=w122:T15, "[[Multiple Decays Fit Parameters]]"=w119:dbl[][], "[Decay Fit Parameter Names]"=w118:T1[], "[[Average Lifetimes]]"=w100:dbl[][])  [unwired: 3 out]
        n21 = property class="ImageControl"(reference=w142, error in=w139) -> (error out=w55:errorcluster, "ROI"=w133:T52)  [unwired: 1 out]
        n22 = call "Alligator Variables Storage.vi"("AlliGator Variable"=AlliGator_Variables_List."Files:Dataset Channel" ("Alligator Variable"), "Error In"=w55) -> ("Error Out"=w97:errorcluster, "Data out"=w99:variant)  [unwired: 7 in, 1 out]
        n23 = call-poly "Variant to Data.vi"("Variant"=w99) -> ("U16 Value"=w96:u16)  [unwired: 8 in]
        n24 = Format Into String(error in=w97, w71) -> (resulting string=w82:string, error out=w73:errorcluster)  [unwired: 2 in]
        n25 = case shown="1" w96 {
          tunnel: [w510 w512] -> w116
          tunnel: w114 -> [_ w512]
          tunnel: [w509 w511] -> w95
          tunnel: w115 -> [_ w511]
          tunnel: w113 -> [w510 _]
          tunnel: w112 -> [w509 _]
          frame 0, Default {
          }
          frame 1 {
          }
        }
        n26 = Search 1D Array(1D array=w118, element=w71) -> (index of element=w121:i32)  [unwired: 1 in]
        n27 = call "Alligator Variables Storage.vi"("Get(F)/Set"=TRUE, "AlliGator Variable"=AlliGator_Variables_List."Image Profile:Plotted Fit Parameter" ("Alligator Variable"), "Error In"=w73, "Data in"=w71) -> ("Error Out"=w72:errorcluster)  [unwired: 5 in, 2 out]
        n28 = case shown="True" w68 {
          tunnel: w62 -> [w528 _]
          tunnel: [w528 w533] -> w86
          tunnel: w125 -> [_ w535]
          tunnel: w116 -> [_ w534]
          tunnel: w124 -> [_ w532]
          tunnel: w95 -> [_ w531]
          tunnel: w123 -> [_ w530]
          tunnel: w122 -> [_ w529]
          frame False {
          }
          frame True {
            n29 = case shown="\"Single Gate\"" w535 {
              tunnel: w534 -> [_ _ _ w542]
              tunnel: [w536 w540 w541 w542] -> w533
              tunnel: w532 -> [w538 _ _ _]
              tunnel: w531 -> [w539 _ _ _]
              tunnel: w530 -> [_ w540 _ _]
              tunnel: w529 -> [_ _ w541 _]
              frame "Single Gate" {
                n30 = Decrement(x=w538) -> (x-1=w537:u16)
                n31 = Index Array(array=w539, index=w537) -> (element=w536:T15)
              }
              frame "White Ligth Image" {
              }
              frame "Mask Image" {
              }
              frame "Sum of All Gates", Default {
              }
            }
          }
        }
        n32 = call "AlliGator Settings Storage.vi"("AlliGator Settings List"=AlliGator_Settings_List."Phasor Plot:Phasor Ratio Color-Coded Quantity", "Error In"=w72) -> ("Error Out"=w106:errorcluster, "Variant Data out"=w104:variant)  [unwired: 8 in]
        n33 = Variant To Data(error in=w106, type=AlliGator_Phasor_Ratio_Color-Coded_Quantity."Phasor Ratio (f1 or a1)" ("Displayed Quantity"), Variant=w104) -> (data=w102:T12, error out=w105:errorcluster)
        n34 = Unbundle By Name(w133) -> ("Contours"=w132:T53)
        n35 = case shown="0, Default" w121 {
          selector: w121 -> [w521 _]
          tunnel: w116 -> [w520 _]
          tunnel: w119 -> [w519 _]
          tunnel: [w516 _] -> w120
          tunnel: w55 -> [w518 w527]
          tunnel: [w515 w527] -> w54
          tunnel: w53 -> [w513 _]
          frame 0, Default {
            n36 = call "IMAQ GetImageInfo"("error in (no error)"=w518, "Image"=w520) -> ("error out"=w526:errorcluster, "Y Resolution"=w525:i32, "X Resolution"=w524:i32)  [unwired: 2 in, 5 out]
            n37 = Compound Arithmetic op=ADD(w521, 2 ("value")) -> (w523:i32)
            n38 = call "AlliGator Get Decay Fit Parameter Map Data.vi"("Multiple Decays Fit Parameters"=w519, "Compute Decay Fit Parameter Map"=TRUE, "Output ROI centers?"=FALSE, "X Resolution"=w524, "Y Resolution"=w525, "Error In"=w526, "Map index"=w523, "Selected ROI Array"=w513) -> ("Map Data (V x H)"=w516:dbl[][], "Error Out"=w515:errorcluster)  [unwired: 3 in, 3 out]
          }
          frame ..-1 {
          }
        }
        n39 = Array Size(array=w95) -> (size(s)=w93:i32)
        n40 = Equal?(x=w102, y=AlliGator_Phasor_Ratio_Color-Coded_Quantity."Phasor Ratio (f1 or a1)") -> (x = y?=w81:bool)
        n41 = Index Array(array=w132) -> (element=w131:T54)  [unwired: 1 in]
        n42 = call "AlliGator Settings Storage.vi"("AlliGator Settings List"=AlliGator_Settings_List."Phasor Graph:Phasor Ratio Type", "Error In"=w105) -> ("Error Out"=w108:errorcluster, "Variant Data out"=w109:variant)  [unwired: 8 in]
        n43 = Unbundle By Name(w131) -> ("ROI Type"=w129:u32, "Points"=w130:i32[])
        n44 = Variant To Data(error in=w108, type=w110, Variant=w109) -> (data=w111:T13)  [unwired: 1 out]
        n45 = Equal?(x=w110, y=w111) -> (x = y?=w80:bool)
        n46 = Coerce To Type(0:w129, 1:Image_ROI_Type."No Selection" ("ROI Type")) -> (2:w57:T9)
        n47 = Compound Arithmetic op=MULTIPLY(w93, w135) -> (w94:dbl)
        n48 = call "AlliGator Phasor Frequency.vi"() -> ("Phasor Frequency"=w127:dbl[unit])
        n49 = case shown="\"Polygon\", \"Broken Line\"" w57 {
          selector: w57 -> [_ w152 _ _ _]
          tunnel: w54 -> [w144 w175 w300 w350 w465]
          tunnel: [w144 w146 w286 w335 w456] -> w61
          tunnel: w130 -> [_ w148 w285 w364 w478]
          tunnel: [_ w169 w299 w361 w477] -> w92
          tunnel: w126 -> [_ w168 w303 w363 w474]
          tunnel: w127 -> [_ w167 w302 w362 w473]
          tunnel: [_ w151 w289 w353 w462] -> w91
          tunnel: w86 -> [_ w163 w298 w360 w472]
          tunnel: [_ w160 w296 w359 w471] -> w90
          tunnel: w120 -> [_ w159 w295 w358 w470]
          tunnel: [_ w157 w294 w357 w469] -> w89
          tunnel: w80 -> [_ w155 w293 w356 w468]
          tunnel: w100 -> [_ w154 w292 w355 w467]
          tunnel: w81 -> [_ w153 w291 w354 w466]
          tunnel: w67 -> [_ w150 w288 w349 w461]
          tunnel: w94 -> [_ w149 w287 w348 w460]
          tunnel: w65 -> [_ _ _ w347 _]
          tunnel: [_ _ _ w345 _] -> w63
          tunnel: w84 -> [_ _ _ w343 _]
          tunnel: [_ _ _ w341 _] -> w79
          tunnel: [_ _ _ w340 _] -> w78
          tunnel: [_ _ _ w339 _] -> w77
          tunnel: w66 -> [_ _ _ w338 _]
          tunnel: [_ _ _ w337 _] -> w64
          tunnel: [_ w145 w279 w332 w458] -> w56
          frame "No Selection", Default {
          }
          frame "Polygon", "Broken Line" {
            # "leftover vertices"
            # "first vertex"
            n50 = Array Size(array=w148) -> (size(s)=w174:i32)
            n51 = Quotient & Remainder(x=w174, y=2) -> (floor(x/y)=w173:i32)  [unwired: 1 out]
            n52 = for "For a multi-segment line, read individual segments" {
              N: w173 -> [_]
              shift-right: [w217] -> w147
              shift-left: w175 -> [w218]
              tunnel: [w215] -> w171 mode=concatenating if=w198
              tunnel: [w214] -> w170
              shift-right: [w210] -> _
              shift-left: w148 -> [w213]
              shift-right: [w208] -> _
              shift-left: _ -> [w207]
              tunnel: w168 -> [w206]
              tunnel: w167 -> [w205]
              tunnel: [w204] -> w166 mode=concatenating if=w198
              tunnel: [w203] -> w164
              tunnel: w163 -> [w216]
              tunnel: [w202] -> w162 mode=concatenating if=w198
              tunnel: [w201] -> w161
              tunnel: w159 -> [w200]
              tunnel: [w199] -> w158 mode=concatenating if=w198
              tunnel: [w197] -> w156
              tunnel: w155 -> [w196]
              tunnel: w154 -> [w195]
              tunnel: w153 -> [w194]
              tunnel: w150 -> [w193]
              tunnel: w149 -> [w192]
              i -> [w211]
              n53 = Split 1D Array(array=w213, index=2) -> (first subarray=w209:i32[], second subarray=w210:i32[])
              n54 = case shown="1, Default" w211 {
                tunnel: w218 -> [w219 w236]
                tunnel: [w219 w246] -> w217
                tunnel: w216 -> [_ w237]
                tunnel: [_ w250] -> w215
                tunnel: [_ w249] -> w214
                tunnel: w209 -> [w220 w223]
                tunnel: [w220 w223] -> w208
                tunnel: w207 -> [_ w224]
                tunnel: [_ TRUE] -> w198
                tunnel: w206 -> [_ w244]
                tunnel: w205 -> [_ w243]
                tunnel: [_ w241] -> w204
                tunnel: [_ w240] -> w203
                tunnel: [_ w233] -> w202
                tunnel: [_ w232] -> w201
                tunnel: w200 -> [_ w231]
                tunnel: [_ w229] -> w199
                tunnel: [_ w228] -> w197
                tunnel: w196 -> [_ w227]
                tunnel: w195 -> [_ w225]
                tunnel: w194 -> [_ w226]
                tunnel: w193 -> [_ w222]
                tunnel: w192 -> [_ w221]
                frame 0 {
                  # "preserves the previous point"
                }
                frame 1, Default {
                  n55 = Build Array (concatenate)(w224, w223) -> (w247:i32[])
                  n56 = call "ROI Segment Points to Array of Pixels.vi"("error in (no error)"=w236, "Segment ROI Points"=w247) -> ("Error Out"=w235:errorcluster, "Pixels of the Segment"=w245:cluster{"X":i32, "Y":i32}[])  [unwired: 7 in, 1 out]
                  n57 = for {
                    tunnel: w245 -> [w274] mode=indexing
                    tunnel: w244 -> [w264]
                    tunnel: w243 -> [w263]
                    tunnel: [w273] -> w242 mode=indexing
                    tunnel: [w270] -> w239 mode=indexing
                    tunnel: [w253] -> w238 mode=indexing
                    tunnel: w235 -> [w268]
                    tunnel: w237 -> [w271]
                    tunnel: [w260] -> w234 mode=indexing
                    tunnel: w231 -> [w267]
                    tunnel: [w266] -> w230 mode=indexing
                    tunnel: w227 -> [w258]
                    tunnel: w225 -> [w257]
                    tunnel: w226 -> [w259]
                    tunnel: w222 -> [w252]
                    tunnel: w221 -> [w251]
                    n58 = Unbundle(w274) -> ("X"=w255:i32, "Y"=w256:i32)
                    n59 = Index Array(array=w267, index (row)=w256, index (col)=w255) -> (element=w266:dbl)
                    n60 = Index Array(array=w264, index (row)=w256, index (col)=w255) -> (element=w265:csg)
                    n61 = call "IMAQ Get Pixel Value Wrapper.vi"("Error In"=w268, "Y Coordinate"=w256, "X Coordinate"=w255, "Image"=w271) -> ("Error Out"=w272:errorcluster, "Pixel Value"=w254:sgl)  [unwired: 5 in, 1 out]
                    n62 = call "AlliGator Get Phase Lifetime & Phasor Ratio at Pixel.vi"("error in (no error)"=w268, "Intensity (F)/Amplitude (T) weighted"=w258, "Phasor Frequency"=w263, "Phasor"=w265) -> ("error out"=w269:errorcluster, "Phasor/Amplitude Ratio"=w261:dbl, "Phase Lifetime"=w273:dbl[unit])  [unwired: 4 in, 1 out]
                    n63 = case shown="True" w252 {
                      tunnel: w254 -> [w275 w278]
                      tunnel: [w275 w277] -> w253
                      tunnel: w251 -> [_ w276]
                      frame False {
                      }
                      frame True {
                        # "Bkgd subtraction"
                        n64 = Compound Arithmetic op=ADD(invert w276, w278) -> (w277:dbl)
                      }
                    }
                    n65 = Index Array(array=w257, index (row)=w256, index (col)=w255) -> (element=w262:dbl)
                    n66 = Select(t=w261, s=w259, f=w262) -> (s? t:f=w260:dbl)
                    n67 = Merge Errors(w272, w269) -> (w270:errorcluster)
                  }
                  n68 = Delete From Array(array=w230) -> (deleted portion=w228:dbl, array with subset deleted=w229:dbl[])  [unwired: 2 in]
                  n69 = Delete From Array(array=w238) -> (deleted portion=w249:dbl, array with subset deleted=w250:dbl[])  [unwired: 2 in]
                  n70 = Delete From Array(array=w234) -> (deleted portion=w232:dbl, array with subset deleted=w233:dbl[])  [unwired: 2 in]
                  n71 = Delete From Array(array=w242) -> (deleted portion=w240:dbl[unit], array with subset deleted=w241:dbl[unit][])  [unwired: 2 in]
                  n72 = Merge Errors(w239) -> (w246:errorcluster)
                }
              }
            }
            n73 = case shown="\"Broken Line\"" w152 {
              tunnel: w171 -> [w179 w191]
              tunnel: w170 -> [_ w190]
              tunnel: [w179 w189] -> w169
              tunnel: w166 -> [w178 w188]
              tunnel: [w178 w187] -> w165
              tunnel: w164 -> [_ w186]
              tunnel: w162 -> [w177 w185]
              tunnel: w161 -> [_ w184]
              tunnel: [w177 w183] -> w160
              tunnel: w158 -> [w176 w182]
              tunnel: [w176 w181] -> w157
              tunnel: w156 -> [_ w180]
              frame "Polygon", Default {
              }
              frame "Broken Line" {
                n74 = Build Array (concatenate)(w191, w190) -> (w189:dbl[])
                n75 = Build Array (concatenate)(w188, w186) -> (w187:dbl[unit][])
                n76 = Build Array (concatenate)(w185, w184) -> (w183:dbl[])
                n77 = Build Array (concatenate)(w182, w180) -> (w181:dbl[])
              }
            }
            n78 = call "First & Last Point.vi"("Error In"=w147, "Point Coordinates Array"=w148) -> ("Error Out"=w146:errorcluster, "First & Last Point"=w145:cluster{"X":i32, "Y":i32}[])  [unwired: 8 in]
            n79 = node(w165) -> (w151:dbl[])
          }
          frame "Line" {
            n80 = call "ROI Segment Points to Array of Pixels.vi"("error in (no error)"=w300, "Segment ROI Points"=w285) -> ("Error Out"=w297:errorcluster, "Pixels of the Segment"=w284:cluster{"X":i32, "Y":i32}[])  [unwired: 7 in, 1 out]
            n81 = Array Size(array=w284) -> (size(s)=w283:i32)
            n82 = Decrement(x=w283) -> (x-1=w282:i32)
            n83 = Index Array(array=w284, index #2=w282) -> (element #1=w281:cluster{"X":i32, "Y":i32}, element #2=w280:cluster{"X":i32, "Y":i32})  [unwired: 1 in]
            n84 = for {
              tunnel: w303 -> [w318]
              tunnel: w284 -> [w327] mode=indexing
              tunnel: w302 -> [w316]
              tunnel: [w319] -> w290 mode=indexing
              tunnel: w298 -> [w326]
              tunnel: w297 -> [w321]
              tunnel: [w324] -> w301 mode=indexing
              tunnel: [w306] -> w299 mode=indexing
              tunnel: [w311] -> w296 mode=indexing
              tunnel: w295 -> [w323]
              tunnel: [w322] -> w294 mode=indexing
              tunnel: w293 -> [w315]
              tunnel: w292 -> [w310]
              tunnel: w291 -> [w314]
              tunnel: w288 -> [w305]
              tunnel: w287 -> [w304]
              n85 = Unbundle(w327) -> ("X"=w309:i32, "Y"=w308:i32)
              n86 = call "IMAQ Get Pixel Value Wrapper.vi"("Error In"=w321, "Y Coordinate"=w308, "X Coordinate"=w309, "Image"=w326) -> ("Error Out"=w325:errorcluster, "Pixel Value"=w307:sgl)  [unwired: 5 in, 1 out]
              n87 = Index Array(array=w323, index (row)=w308, index (col)=w309) -> (element=w322:dbl)
              n88 = Index Array(array=w310, index (row)=w308, index (col)=w309) -> (element=w313:dbl)
              n89 = Index Array(array=w318, index (row)=w308, index (col)=w309) -> (element=w317:csg)
              n90 = call "AlliGator Get Phase Lifetime & Phasor Ratio at Pixel.vi"("error in (no error)"=w321, "Intensity (F)/Amplitude (T) weighted"=w315, "Phasor Frequency"=w316, "Phasor"=w317) -> ("error out"=w320:errorcluster, "Phasor/Amplitude Ratio"=w312:dbl, "Phase Lifetime"=w319:dbl[unit])  [unwired: 4 in, 1 out]
              n91 = case shown="True" w305 {
                tunnel: w307 -> [w328 w331]
                tunnel: [w328 w330] -> w306
                tunnel: w304 -> [_ w329]
                frame False {
                }
                frame True {
                  # "Bkgd subtraction"
                  n92 = Compound Arithmetic op=ADD(invert w329, w331) -> (w330:dbl)
                }
              }
              n93 = Select(t=w312, s=w314, f=w313) -> (s? t:f=w311:dbl)
              n94 = Merge Errors(w325, w320) -> (w324:errorcluster)
            }
            n95 = Build Array(w281, w280) -> (w279:cluster{"X":i32, "Y":i32}[])
            n96 = Merge Errors(w301) -> (w286:errorcluster)
            n97 = node(w290) -> (w289:dbl[])
          }
          frame "Rectangle", "Rotated Rectangle" {
            n98 = Not(x=w343) -> (.not. x?=w342:bool)
            n99 = call "Convert Rectangle Data to Segment Array v2.vi"("Error In"=w350, "Box Profile Type"=w347, "(Rotated) Rectangle Data"=w364) -> ("Error Out"=w334:errorcluster, "Median End Points"=w333:cluster{"X":dbl, "Y":dbl}[], "Rectange Profile Segments"=w352:cluster{"Segment ROI Points":i32[]}[], "Number of Points"=w344:i32)  [unwired: 4 in, 1 out]
            n100 = for "For Loop on perpendicular strips" {
              tunnel: w352 -> [w409] mode=indexing
              tunnel: w363 -> [w408]
              tunnel: w362 -> [w406]
              tunnel: [w392] -> w351 mode=indexing
              tunnel: w334 -> [w404]
              tunnel: [w382] -> w361 mode=indexing
              tunnel: w360 -> [w403]
              tunnel: [w394] -> w359 mode=indexing
              tunnel: w358 -> [w401]
              tunnel: [w388] -> w357 mode=indexing
              tunnel: w356 -> [w400]
              tunnel: w355 -> [w399]
              tunnel: w354 -> [w398]
              tunnel: [w393] -> w353 mode=indexing
              tunnel: w349 -> [w384]
              tunnel: w348 -> [w383]
              tunnel: [w381] -> w336
              tunnel: w342 -> [w368]
              tunnel: [w374] -> w341 mode=indexing
              tunnel: [w373] -> w340 mode=indexing
              tunnel: [w372] -> w339 mode=indexing
              tunnel: w338 -> [w371]
              tunnel: [w365] -> w337 mode=indexing
              n101 = Unbundle(w409) -> ("Segment ROI Points"=w386:i32[])
              n102 = call "ROI Segment Points to Array of Pixels.vi"("error in (no error)"=w404, "Segment ROI Points"=w386) -> ("Error Out"=w402:errorcluster, "Number of Points"=w381:i32, "Pixels of the Segment"=w407:cluster{"X":i32, "Y":i32}[])  [unwired: 7 in]
              n103 = for "For Loop on strip pixels" {
                tunnel: w408 -> [w442]
                tunnel: w407 -> [w451] mode=indexing
                tunnel: w406 -> [w440]
                tunnel: [w443] -> w397 mode=indexing if=w426
                tunnel: w403 -> [w450]
                tunnel: w402 -> [w445]
                tunnel: [w448] -> w405 mode=indexing
                tunnel: [w429] -> w385 mode=indexing if=w426
                tunnel: [w435] -> w395 mode=indexing if=w426
                tunnel: w401 -> [w447]
                tunnel: [w446] -> w389 mode=indexing if=w426
                tunnel: w400 -> [w439]
                tunnel: w399 -> [w434]
                tunnel: w398 -> [w438]
                tunnel: w384 -> [w431]
                tunnel: w383 -> [w430]
                n104 = Unbundle(w451) -> ("X"=w433:i32, "Y"=w432:i32)
                n105 = call "IMAQ Get Pixel Value Wrapper.vi"("Error In"=w445, "Y Coordinate"=w432, "X Coordinate"=w433, "Image"=w450) -> ("Error Out"=w449:errorcluster, "Pixel Value"=w428:sgl)  [unwired: 5 in, 1 out]
                n106 = Index Array(array=w447, index (row)=w432, index (col)=w433) -> (element=w446:dbl)
                n107 = Index Array(array=w434, index (row)=w432, index (col)=w433) -> (element=w437:dbl)
                n108 = Index Array(array=w442, index (row)=w432, index (col)=w433) -> (element=w441:csg)
                n109 = call "AlliGator Get Phase Lifetime & Phasor Ratio at Pixel.vi"("error in (no error)"=w445, "Intensity (F)/Amplitude (T) weighted"=w439, "Phasor Frequency"=w440, "Phasor"=w441) -> ("error out"=w444:errorcluster, "Phasor/Amplitude Ratio"=w436:dbl, "Phase Lifetime"=w443:dbl[unit])  [unwired: 4 in, 1 out]
                n110 = Not A Number/Path/Refnum?(number/path/refnum=w428) -> (NaN/Path/Refnum?=w427:bool)
                n111 = case shown="True" w431 {
                  tunnel: w428 -> [w452 w455]
                  tunnel: [w452 w454] -> w429
                  tunnel: w430 -> [_ w453]
                  frame False {
                  }
                  frame True {
                    # "Bkgd subtraction"
                    n112 = Compound Arithmetic op=ADD(invert w453, w455) -> (w454:dbl)
                  }
                }
                n113 = Select(t=w436, s=w438, f=w437) -> (s? t:f=w435:dbl)
                n114 = Not(x=w427) -> (.not. x?=w426:bool)
                n115 = Merge Errors(w449, w444) -> (w448:errorcluster)
              }
              n116 = Merge Errors(w405) -> (w370:errorcluster)
              n117 = case shown="\"Integrated Intensity\", Default" w371 {
                tunnel: w385 -> [w412 w419 w422]
                tunnel: [w411 w418 w425] -> w382
                tunnel: [_ w417 w424] -> w367
                tunnel: [_ w416 w423] -> w366
                tunnel: w370 -> [w410 w415 w421]
                tunnel: [w410 w414 w420] -> w369
                frame "Integrated Intensity", Default {
                  n118 = Add Array Elements(numeric array=w412) -> (sum=w411:dbl)
                }
                frame "Average Intensity" {
                  n119 = call "Weighted Array Mean & SDV.vi"("Error In"=w415, "Weight Array"=dbl[] [], "Array"=w419) -> ("Error Out"=w414:errorcluster, "SDV (weighted)"=w416:dbl, "SDV (classic)"=w417:dbl, "Average Value (weighted)"=w418:dbl)  [unwired: 3 in, 2 out]
                }
                frame "Intensity-weighted Average Intensity" {
                  n120 = call "Weighted Array Mean & SDV.vi"("Error In"=w421, "Weight Array"=w422, "Array"=w422) -> ("Error Out"=w420:errorcluster, "SDV (weighted)"=w423:dbl, "SDV (classic)"=w424:dbl, "Average Value (weighted)"=w425:dbl)  [unwired: 3 in, 2 out]
                }
              }
              n121 = node(w397) -> (w396:dbl[])
              n122 = call "Weighted Array Mean & SDV.vi"("Error In"=w370, "Weight Array"=w385, "Array"=w396) -> ("Error Out"=w391:errorcluster, "SDV (weighted)"=w379:dbl, "SDV (classic)"=w380:dbl, "Average Value (weighted)"=w393:dbl)  [unwired: 3 in, 2 out]
              n123 = call "Weighted Array Mean & SDV.vi"("Error In"=w370, "Weight Array"=w385, "Array"=w395) -> ("Error Out"=w390:errorcluster, "SDV (weighted)"=w377:dbl, "SDV (classic)"=w378:dbl, "Average Value (weighted)"=w394:dbl)  [unwired: 3 in, 2 out]
              n124 = call "Weighted Array Mean & SDV.vi"("Error In"=w370, "Weight Array"=w385, "Array"=w389) -> ("Error Out"=w387:errorcluster, "SDV (weighted)"=w375:dbl, "SDV (classic)"=w376:dbl, "Average Value (weighted)"=w388:dbl)  [unwired: 3 in, 2 out]
              n125 = Merge Errors(w369, w391, w390, w387) -> (w392:errorcluster)
              n126 = Select(t=w367, s=w368, f=w366) -> (s? t:f=w365:dbl)
              n127 = Select(t=w380, s=w368, f=w379) -> (s? t:f=w374:dbl)
              n128 = Select(t=w378, s=w368, f=w377) -> (s? t:f=w373:dbl)
              n129 = Select(t=w376, s=w368, f=w375) -> (s? t:f=w372:dbl)
            }
            n130 = Merge Errors(w351) -> (w335:errorcluster)
            n131 = To Long Integer(number=w333) -> (32bit integer=w332:cluster{"X":i32, "Y":i32}[])
            n132 = Format Into String(format string=" (L:%d, W:%d)", w344, w336) -> (resulting string=w345:string)  [unwired: 2 in, 1 out]
          }
          frame "Freehand Line" {
            n133 = call "Remove Duplicate Consecutive Vertices.vi"("Error In"=w465, "Freehand Line Points (in)"=w478) -> ("Error Out"=w464:errorcluster, "Freehand Line Points (out)"=w459:i32[])  [unwired: 8 in]
            n134 = Decimate 1D Array(w459) -> (w476:i32[], w475:i32[])
            n135 = for {
              tunnel: w476 -> [w485] mode=indexing
              tunnel: [w482] -> w477 mode=indexing
              tunnel: w475 -> [w484] mode=indexing
              tunnel: w473 -> [w493]
              tunnel: [w496] -> w463 mode=indexing
              tunnel: w474 -> [w494]
              tunnel: w472 -> [w501]
              tunnel: w464 -> [w497]
              tunnel: [w500] -> w479 mode=indexing
              tunnel: [w489] -> w471 mode=indexing
              tunnel: w470 -> [w486]
              tunnel: [w499] -> w469 mode=indexing
              tunnel: w468 -> [w488]
              tunnel: w467 -> [w487]
              tunnel: w466 -> [w492]
              tunnel: w461 -> [w481]
              tunnel: w460 -> [w480]
              n136 = Index Array(array=w494, index (row)=w484, index (col)=w485) -> (element=w495:csg)
              n137 = Index Array(array=w487, index (row)=w484, index (col)=w485) -> (element=w490:dbl)
              n138 = call "IMAQ Get Pixel Value Wrapper.vi"("Error In"=w497, "Y Coordinate"=w484, "X Coordinate"=w485, "Image"=w501) -> ("Error Out"=w502:errorcluster, "Pixel Value"=w483:sgl)  [unwired: 5 in, 1 out]
              n139 = call "AlliGator Get Phase Lifetime & Phasor Ratio at Pixel.vi"("error in (no error)"=w497, "Intensity (F)/Amplitude (T) weighted"=w488, "Phasor Frequency"=w493, "Phasor"=w495) -> ("error out"=w498:errorcluster, "Phasor/Amplitude Ratio"=w491:dbl, "Phase Lifetime"=w496:dbl[unit])  [unwired: 4 in, 1 out]
              n140 = case shown="True" w481 {
                tunnel: w483 -> [w503 w506]
                tunnel: [w503 w505] -> w482
                tunnel: w480 -> [_ w504]
                frame False {
                }
                frame True {
                  # "Bkgd subtraction"
                  n141 = Compound Arithmetic op=ADD(invert w504, w506) -> (w505:dbl)
                }
              }
              n142 = Select(t=w491, s=w492, f=w490) -> (s? t:f=w489:dbl)
              n143 = Index Array(array=w486, index (row)=w484, index (col)=w485) -> (element=w499:dbl)
              n144 = Merge Errors(w502, w498) -> (w500:errorcluster)
            }
            n145 = Merge Errors(w479) -> (w457:errorcluster)
            n146 = call "First & Last Point.vi"("Error In"=w457, "Point Coordinates Array"=w459) -> ("Error Out"=w456:errorcluster, "First & Last Point"=w458:cluster{"X":i32, "Y":i32}[])  [unwired: 8 in]
            n147 = node(w463) -> (w462:dbl[])
          }
        }
        n148 = call "AlliGator Build Image Profile Plots.vi"("Intensity"=w92, "ROI Type"=w57, "Box Profile Type"=w65, "ROI Size String"=w63, "Phase Lifetime"=w91, "Average Lifetime/Phasor Ratio"=w90, "Fit Parameter"=w89, "Error In"=w61, "Fit Parameter Name"=w82, "ratio(T)/<tau>(F)"=w81, "< t>_I (F)/<t>_A"=w80) -> ("Plot Array"=w88:T10[], "Error Out"=w83:errorcluster)  [unwired: 3 in]
        n149 = call "AlliGator Build Image SDV Profile Plots.vi"("Intensity SDV"=w64, "ROI Type"=w57, "Box Profile Type"=w65, "ROI Size String"=w63, "Phase Lifetime SDV"=w79, "Average Lifetime/Phasor Ratio SDV"=w78, "Fit Parameter SDV"=w77, "Error In"=w83, "Fit Parameter Name"=w82, "ratio(T)/<tau>(F)"=w81, "< t>_I (F)/<t>_A"=w80) -> ("Plot Array"=w76:T10[], "Error Out"=w75:errorcluster)  [unwired: 3 in]
        n150 = Build Array (concatenate)(w88, w76) -> (w59:T10[])
        n151 = Bundle By Name(cluster=T8 {"ROI Type"=enum."No Selection", "End Points"=[{"X"=98.0, "Y"=43.0}, {"X"=133.0, "Y"=78.0}], "Profile Data"=[]} ("Image Profile Data"), "ROI Type"=w57, "End Points"=w56, "Profile Data"=w59) -> (w58:T8)
        n152 = Generate User Event(user event=w140, event data cluster=w58, error in=w75) -> (error out=w87:errorcluster)  [unwired: 1 in, 1 out]
        n153 = in-place-dvr #1() -> (w51:refnum<data-value>, w44:errorcluster)  [unwired: 1 in]
      }
      n154 = Merge Errors(w44, w29) -> (w43:errorcluster)
    }
  }
  "error out" <- w7
  "AlliGator IV DVR out" <- w9
